vi "End communcation.vi"(8 "error in (no error)":errorcluster, 11 "Serial port":refnum<visa-resource-name>) -> (0 "error out":errorcluster, 1 "success":bool, 3 "Serial port out":refnum<visa-resource-name>)   [LabVIEW 2010]
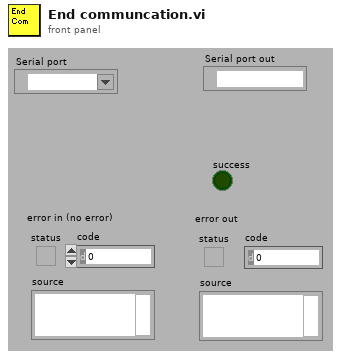
[diagram p1: front panel]
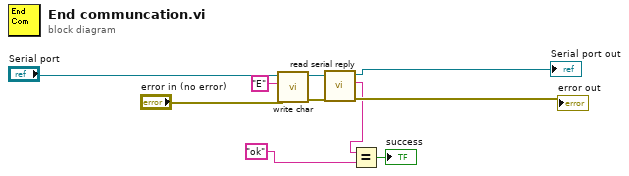
[diagram p0: block diagram]
diagram:
  n1 = call "write char.vi"("error in (no error)"="error in (no error)", "write buffer"="E", "Serial port"="Serial port") -> ("error out"=w6:errorcluster, "Serial Port"=w10:refnum<visa-resource-name>)  [unwired: 6 in, 1 out]
  n2 = call "read serial reply.vi"("error in (no error)"=w6, "Serial Port"=w10) -> ("error out"=→"error out":errorcluster, "reply"=w3:string, "Serial Port out"=→"Serial port out":refnum<visa-resource-name>)  [unwired: 7 in]
  n3 = Equal?(x=w3, y="ok" ("write buffer")) -> (x = y?=→"success":bool)
